vi "R.vizulis 1.vi"() -> ()   [LabVIEW 2022 SP3]
uses:
  <vilib>/Utility/file.llb/Write Delimited Spreadsheet (I64).vi
  <vilib>/Utility/file.llb/Read Delimited Spreadsheet (I64).vi
panel:
  out "all rows":i64[][](array[numeric])
  in  "file path (dialog if empty)":path
  out "Array":dbl[](array[numeric])
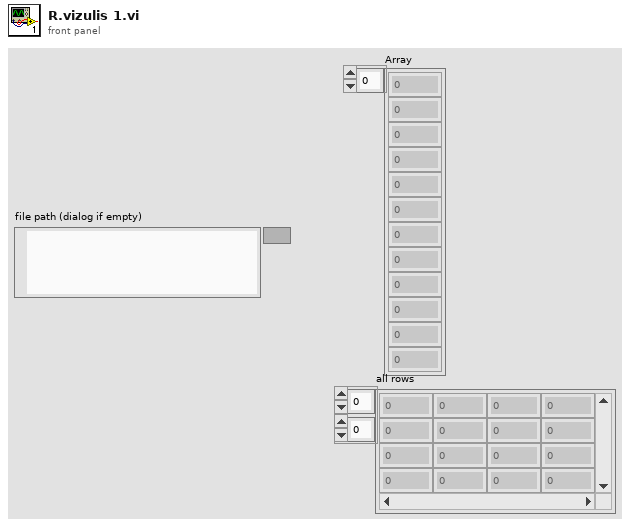
[diagram p1: front panel]
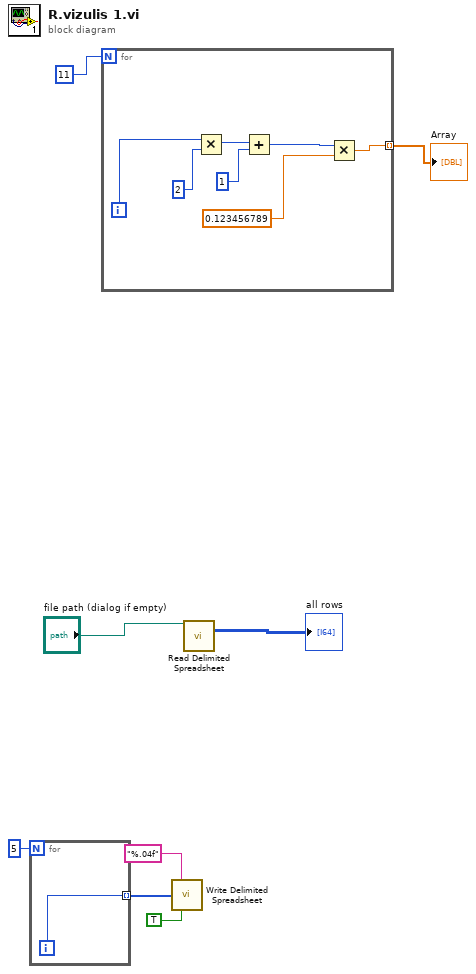
[diagram p0: block diagram]
diagram:
  n1 = for {
    N: 5 -> [_]
    tunnel: [w9] -> w6 mode=indexing
    i -> [w9]
  }
  n2 = for {
    N: 11 -> [_]
    tunnel: [w11] -> w7 mode=indexing
    i -> [w16]
    n3 = Multiply(x=w16, y=2) -> (x*y=w14:i32)
    n4 = Add(x=w14, y=1) -> (x+y=w10:i32)
    n5 = Multiply(x=w10, y=0.123456789) -> (x*y=w11:dbl)
  }
  "Array" <- w7
  n6 = call-poly <vilib>:"Write Delimited Spreadsheet.vi"("format (%d)"="%.04f", "1D data"=w6, "transpose? (no:F)"=TRUE) -> ()  [unwired: 11 in, 2 out]
  n7 = call-poly <vilib>:"Read Delimited Spreadsheet.vi"("file path (dialog if empty)"="file path (dialog if empty)") -> ("all rows"=→"all rows":i64[][])  [unwired: 9 in, 5 out]
